vi "Auton Enum.vi"(11 "Initial State":T1) -> (3 "Initial State 2":T1)   [LabVIEW 2015]
uses:
  AutoStatesTypeDef.ctl
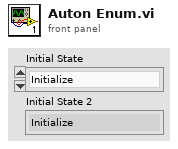
[diagram p1: front panel]
types:
  T1 = typedef "AutoStatesTypeDef.ctl" = enum16{"Initialize", "Line up to shoot", "Align robot", "Drive to goal", "Lower Arms", "Raise Arms", "Drive to defense", "Cross defense", "Turn towards goal", "Shoot", "Retreat", "Stop"}
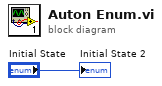
[diagram p0: block diagram]
diagram:
  "Initial State 2" <- "Initial State"
